vi "Destroy.vi"(8 "error in (no error)":errorcluster, 11 "CollapsePanel in":refnum<class "CollapsePanel.lvclass">) -> (0 "error out":errorcluster)   [LabVIEW 2021, in "CollapsePanel.lvclass"]
uses:
  CollapsePanel.lvclass
  CollapsePanel.lvclass/CollapsePanel.ctl
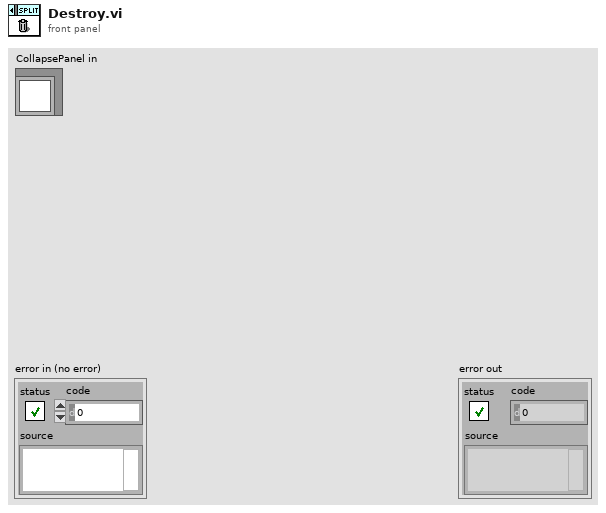
[diagram p1: front panel]
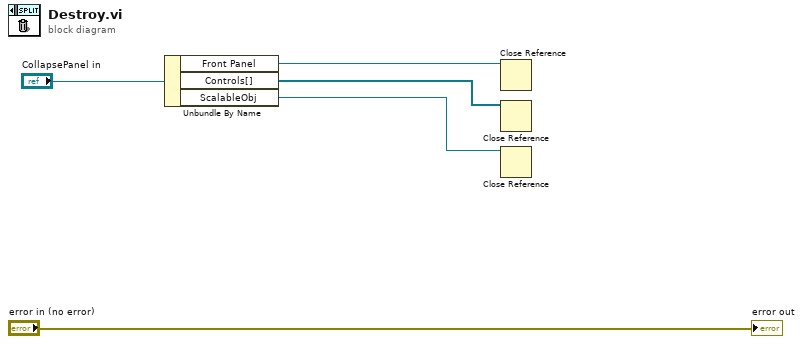
[diagram p0: block diagram]
diagram:
  n1 = Unbundle By Name("CollapsePanel in") -> ("Front Panel"=w4:refnum<vi>, "Controls[]"=w2:refnum<vi>[], "ScalableObj"=w1:refnum<vi>)
  n2 = Close Reference(reference=w4) -> ()  [unwired: 1 in, 1 out]
  n3 = Close Reference(reference=w2) -> ()  [unwired: 1 in, 1 out]
  n4 = Close Reference(reference=w1) -> ()  [unwired: 1 in, 1 out]
  "error out" <- "error in (no error)"
